vi "Get_Current_Scan_client.vi"(0 "ADAM Ch Names":string[](array[string])=["EnFlo Tun:Ultrasonic:Fixed"]) -> (1 "Ch Description Array":T1[](array[typedef]) {"Duty" format="%.0b"; "D" format="%#_5g"; "C" format="%#_5g"; "B" format="%#_5g"; "A" format="%#_5g"}, 2 "String values":string[](array[string]), 3 "Numerical Values":dbl[](array[numeric]) format="%.9f")   [LabVIEW 2011]
uses:
  Sub VIs/ADAM Controls/Ch_description_ADAM.ctl
  Sub VIs/ADAM Controls/Module_type_ADAM.ctl
  Sub VIs/ADAM Controls/Function_ADAM.ctl
  Sub VIs/ADAM Controls/Channel_State.ctl
  Sub VIs/ADAM Controls/Calib_type_ADAM.ctl
  Sub VIs/ADAM Controls/Address.ctl
  Anemometry/Anemometry Sub Vis/Controls/Global_mode.ctl
  Anemometry/Anemometry Sub Vis/Globals/Preference_global.vi
panel:
  in  "server type":refnum<vi>
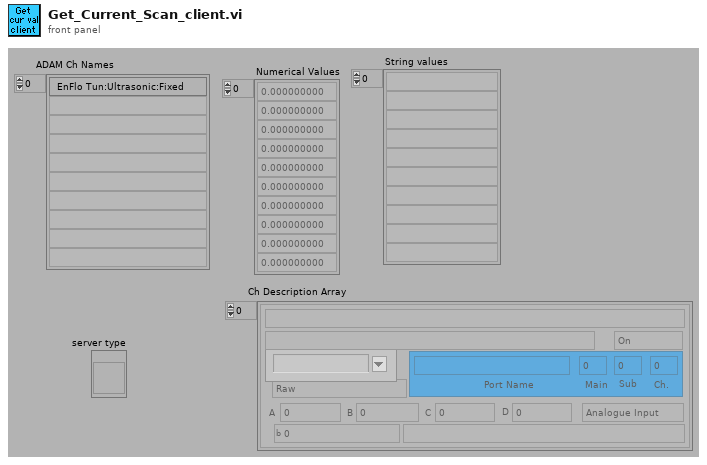
[diagram p1: front panel]
types:
  T1 = typedef "Ch_description_ADAM.ctl" = cluster{"Ch Name":string, "Type":T2, "Function":T3, "Ch State":T4, "Calibration type":T5, "A":dbl, "B":dbl, "C":dbl, "D":dbl, "Comments":string, "Address":T6, "String":string, "Duty":u16}
  T2 = typedef "Module_type_ADAM.ctl" = string
  T3 = typedef "Function_ADAM.ctl" = enum16{"Analogue Input", "Digital Input", "Event counter", "Event rate", "Analogue Output", "Digital Output", "Relay Output"}
  T4 = typedef "Channel_State.ctl" = enum16{"On", "Off", "Always On", "Always Off"}
  T5 = typedef "Calib_type_ADAM.ctl" = enum16{"Raw", "Bx + A", "Cx^2 + Bx + A", "Dx^3 + Cx^2 + Bx + A", "In Band", "Hi-Tec Q", "Hi-Tec M_dot", "Text"}
  T6 = typedef "Address.ctl" = cluster{"Main":i32, "Ch.":i32, "Sub":i32, "Port Name":string}
  T7 = typedef "Server_Comms.ctl" = enum16{"Server Link Healthy", "Do Not Link To Server"}
  T8 = typedef "Global_mode.ctl" = enum16{"Read Global", "Load Global From File", "Write Global to File"}
  T9 = typedef "Update_scan_value.ctl" = cluster{"Channel Name":string, "New Value":dbl}
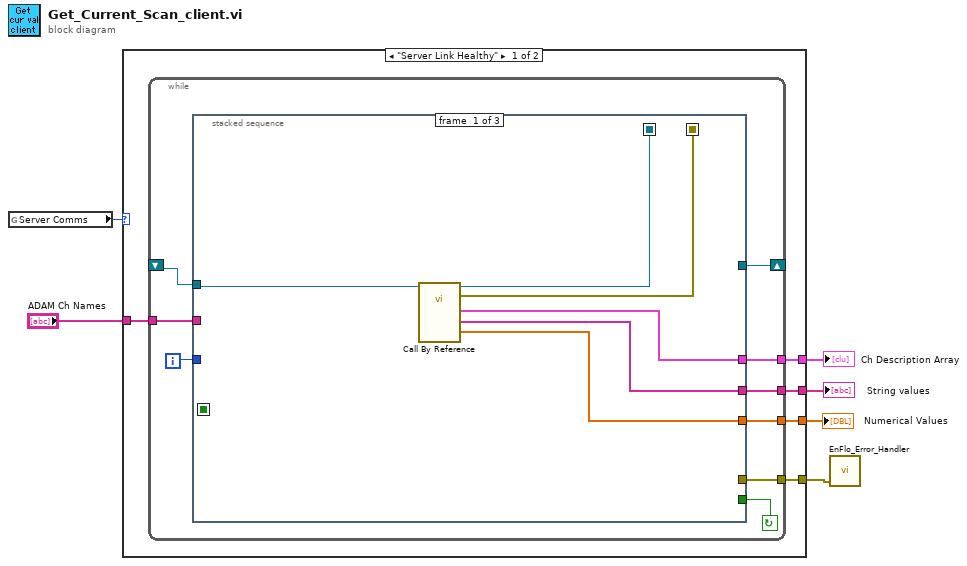
[diagram p0: block diagram]
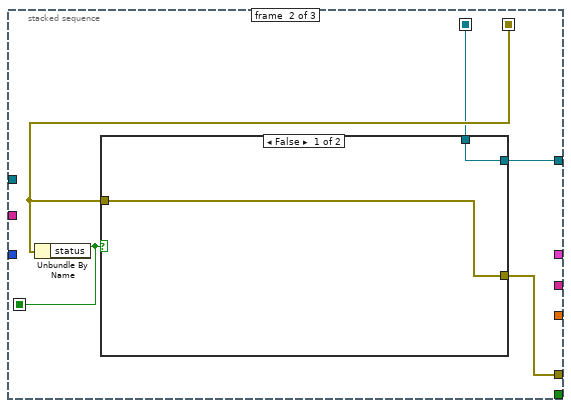
[diagram p2: hidden frame]
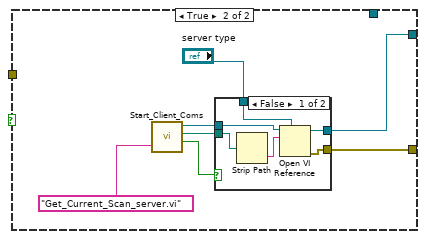
[diagram p3: hidden frame]
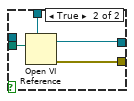
[diagram p4: hidden frame]
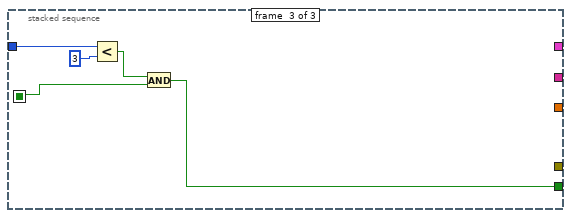
[diagram p5: hidden frame]
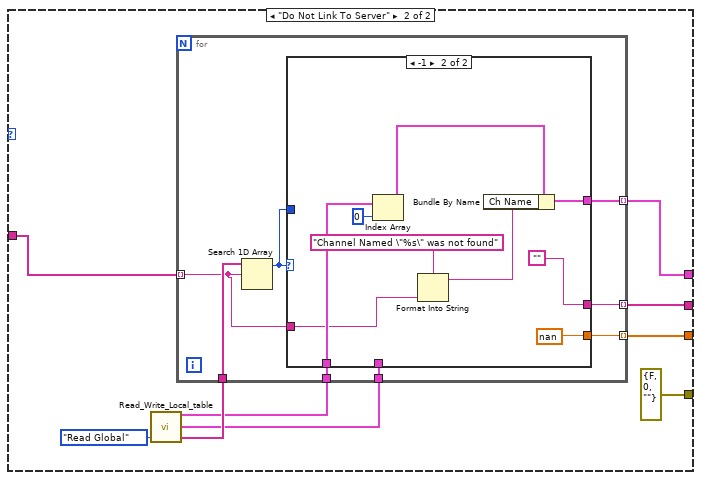
[diagram p6: hidden frame]
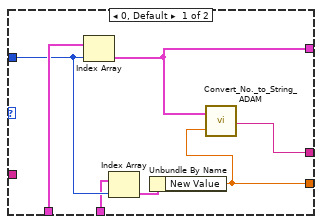
[diagram p7: hidden frame]
diagram:
  n1 = global read "Preference_global.vi" "Server Comms"() -> (w6:T7)
  n2 = case shown="\"Server Link Healthy\"" w6 {
    tunnel: [w11 errorcluster {"status"=FALSE, "code"=0, "source"=""}] -> w5
    tunnel: "ADAM Ch Names" -> [w10 w61]
    tunnel: [w7 w56] -> w1
    tunnel: [w9 w59] -> w3
    tunnel: [w8 w58] -> w2
    frame "Server Link Healthy" {
      n3 = while {
        tunnel: [w13] -> w8
        tunnel: [w14] -> w9
        tunnel: w10 -> [w15]
        tunnel: [w16] -> w11
        shift-left: _ -> [w20]
        shift-right: [w19] -> _
        tunnel: [w12] -> w7
        i -> [w18]
        stop <- w17 continue-if-true
        n4 = stacked-sequence {
          seq-local: [w24 _ _] -> [_ w27 _]
          seq-local: [w26 _ _] -> [_ w28 _]
          seq-local: [_ w30 _] -> [_ _ w52]
          tunnel: w20 -> [w25 _ _]
          tunnel: [_ w31 _] -> w19
          tunnel: w18 -> [_ _ w53]
          tunnel: [_ _ w51] -> w17
          tunnel: [_ w29 _] -> w16
          tunnel: w15 -> [_ _ _]
          tunnel: [w22 _ _] -> w14
          tunnel: [w21 _ _] -> w13
          tunnel: [w23 _ _] -> w12
          frame #0 {
            n5 = call-by-ref "Call By Reference"(reference=w25) -> (reference out=w24:refnum<vi>, error out=w26:errorcluster, "Ch Description Array"=w23:T1[], "String values"=w22:string[], "Numerical Values"=w21:dbl[])  [unwired: 2 in]
          }
          frame #1 {
            n6 = Unbundle By Name(w28) -> ("status"=w30:bool)
            n7 = case shown="False" w30 {
              tunnel: [w32 w36] -> w31
              tunnel: [w33 w34] -> w29
              tunnel: w28 -> [w33 _]
              tunnel: w27 -> [w32 _]
              frame False {
              }
              frame True {
                n8 = call "Start_Client_Coms.vi"("VI name to run on server"="Get_Current_Scan_server.vi") -> ("LabVIEW application reference"=w38:refnum<vi>, "Checked VI name"=w39:path, "Local Call"=w37:bool)  [unwired: 1 in, 1 out]
                n9 = case shown="False" w37 {
                  tunnel: [w44 w50] -> w36
                  tunnel: "server type" -> [w43 w49]
                  tunnel: w39 -> [w42 w48]
                  tunnel: w38 -> [w41 _]
                  tunnel: [w45 w47] -> w34
                  frame False {
                    n10 = Strip Path(path=w42) -> (name=w46:string)  [unwired: 1 out]
                    n11 = Open VI Reference(type specifier VI Refnum (for type only)=w43, application reference (local)=w41, vi path=w46) -> (vi reference=w44:refnum<vi>, error out=w45:errorcluster)  [unwired: 1 in, 2 out]
                  }
                  frame True {
                    n12 = Open VI Reference(type specifier VI Refnum (for type only)=w49, vi path=w48) -> (vi reference=w50:refnum<vi>, error out=w47:errorcluster)  [unwired: 1 in, 3 out]
                  }
                }
              }
            }
          }
          frame #2 {
            n13 = Less?(x=w53, y=3) -> (x < y?=w55:bool)
            n14 = And(x=w55, y=w52) -> (x .and. y?=w51:bool)
          }
        }
      }
    }
    frame "Do Not Link To Server" {
      n15 = call "Read_Write_Local_table.vi"("Mode"=Global_mode."Read Global") -> ("Ch Names"=w62:string[], "Ch Values Out"=w57:T9[], "Channels Descriptions Out"=w60:T1[])  [unwired: 2 in]
      n16 = for {
        tunnel: w62 -> [w72]
        tunnel: w61 -> [w65] mode=indexing
        tunnel: w60 -> [w70]
        tunnel: [w69] -> w56 mode=indexing
        tunnel: [w68] -> w59 mode=indexing
        tunnel: [w67] -> w58 mode=indexing
        tunnel: w57 -> [w66]
        n17 = Search 1D Array(1D array=w72, element=w65) -> (index of element=w71:i32)  [unwired: 1 out]
        n18 = case shown="-1" w71 {
          tunnel: w71 -> [w78 _]
          tunnel: w70 -> [w79 w87]
          tunnel: [w75 w85] -> w69
          tunnel: [w73 ""] -> w68
          tunnel: [w74 nan] -> w67
          tunnel: w66 -> [w77 _]
          tunnel: w65 -> [_ w82]
          frame 0, Default {
            n19 = Index Array(array=w79, index=w78) -> (element=w75:T1)
            n20 = Index Array(array=w77, index=w78) -> (element=w76:T9)
            n21 = Unbundle By Name(w76) -> ("New Value"=w74:dbl)
            n22 = call "Convert_No._to_String_ADAM.vi"("Input number"=w74, "Ch Description"=w75) -> ("Output sting"=w73:string)
          }
          frame -1 {
            n23 = Index Array(array=w87, index=0 ("Index")) -> (element=w86:T1)
            n24 = Format Into String(format string="Channel Named \"%s\" was not found" ("Format String"), w82) -> (resulting string=w80:string)  [unwired: 2 in, 1 out]
            n25 = Bundle By Name(cluster=w86, "Ch Name"=w80) -> (w85:T1)
          }
        }
      }
    }
  }
  "Ch Description Array" <- w1
  "String values" <- w3
  "Numerical Values" <- w2
  n26 = call "EnFlo_Error_Handler.vi"("error in (no error)"=w5) -> ()  [unwired: 2 in, 3 out]
